vi "Monitor.vi"() -> ()   [LabVIEW 2015]
uses:
  Libraries/NI-DAQ/NI-DAQ digitizer parameters.ctl
  Libraries/File/Controls/File formats.ctl
panel:
  out "Shot data":string
  out "file path out":path
  out "Waveform Graph":waveform(dbl)[](graph)
  in  "Shots file":path=path "Y:/ShotHistory2016.txt"
  in  "Log file folder":path=path "C:/Data"
  out "Match out":errorcluster
  out "new path":path
  in  "Root Data Folder":path=path "C:/Data/idot"
  out "File count":i32
  out "New data file event":path
  out "Final error out":errorcluster
  out "Recorder Error Out":errorcluster
  in  "Parameters":T1={"physical channels"="Dev1/ai0:7", "input terminal configuration"=10106, "Range"=10.0, "Sample rate"=1000000.0, "samples per channel"=102400, "Trigger source"="/Dev1/PFI0", "pretrigger samples per channel"=1000, "task"="", "Sample mode"=10178, "Retriggerable"=FALSE, "File Path"=path "C:/Data/idot/test.tdms"} {"Sample mode" items=["Finite Samples"=10178, "Continuous Samples"=10123, "Hardware Timed Single Point"=12522]; "samples per channel" format="%d (0x%x)"; "Sample rate" format="%.2p"; "input terminal configuration" items=["default"=-1, "RSE"=10083, "NRSE"=10078, "Differential"=10106, "Pseudodifferential"=12529]}
  in  "Process Stop Button":bool
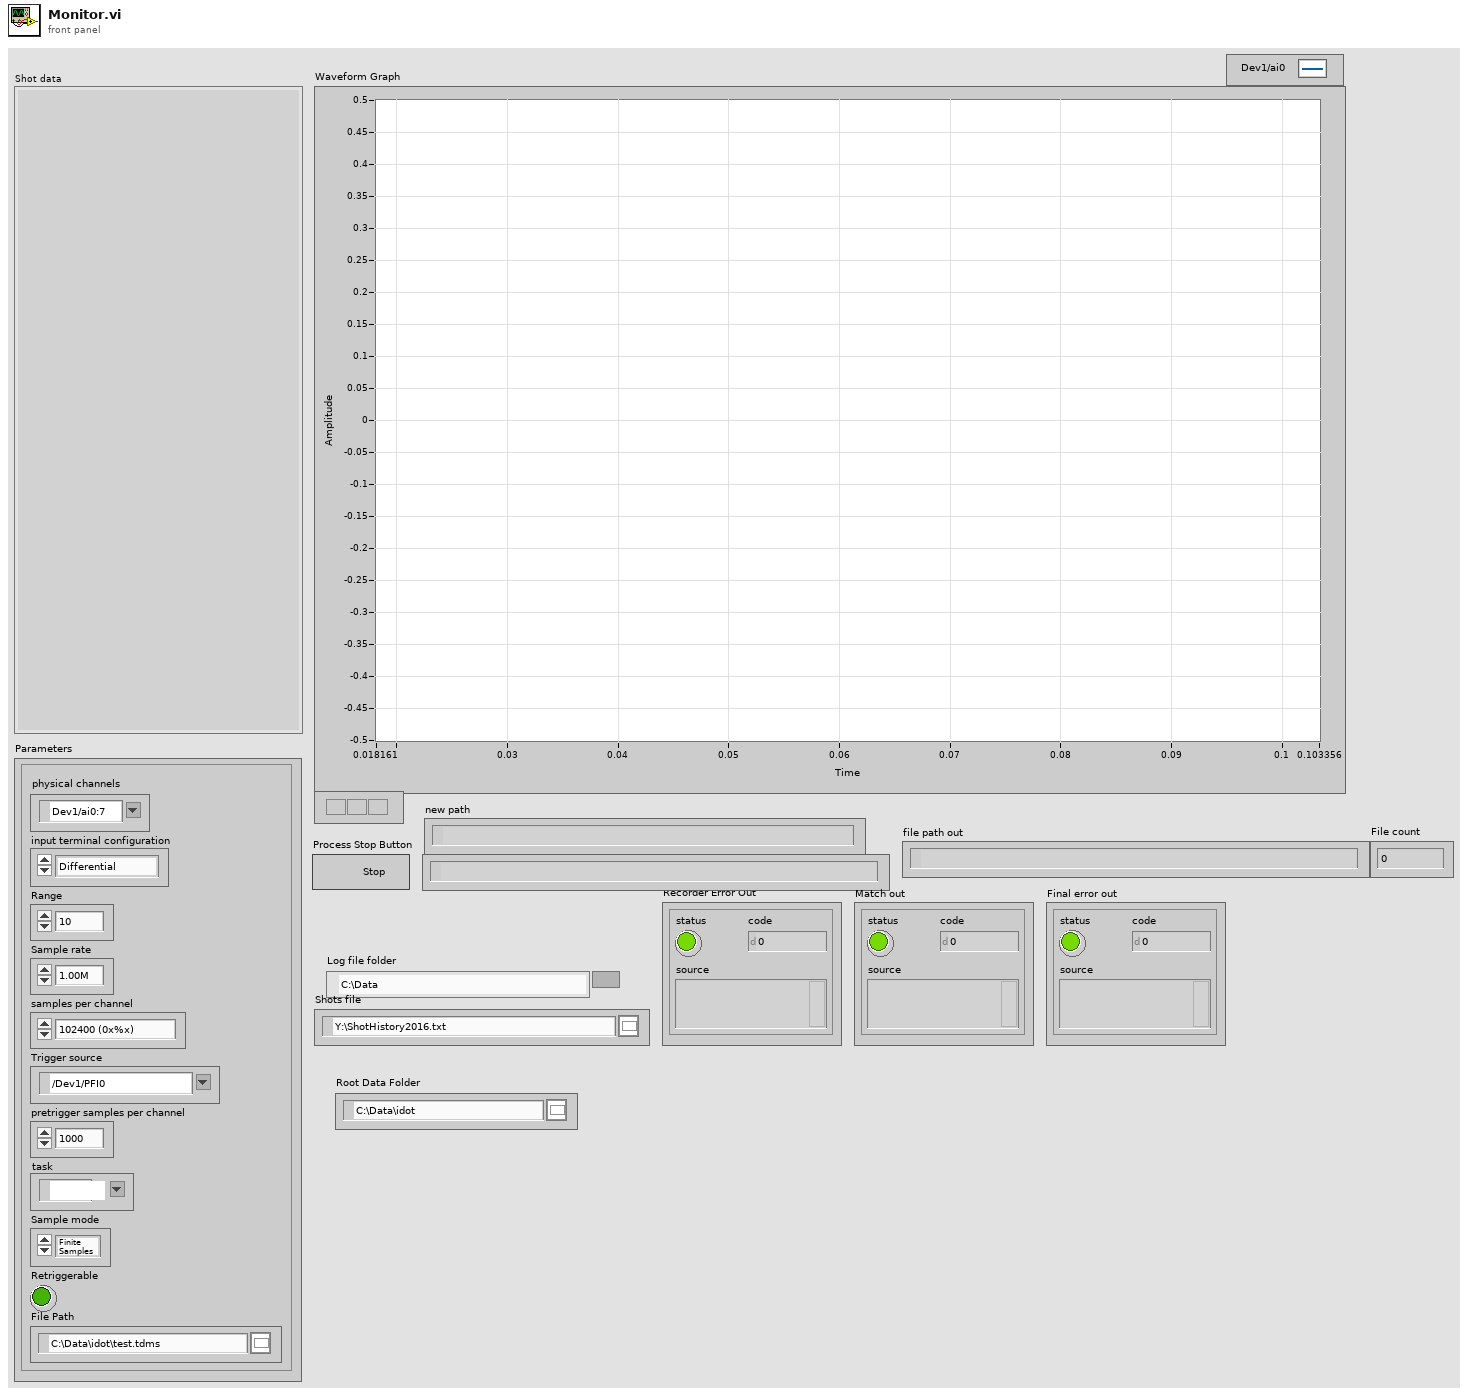
[diagram p1: front panel]
types:
  T1 = typedef "NI-DAQ digitizer parameters.ctl" = cluster{"physical channels":tag, "input terminal configuration":i32, "Range":dbl, "Sample rate":dbl, "samples per channel":i32, "Trigger source":tag, "pretrigger samples per channel":u32, "task":refnum<k21>, "Sample mode":i32, "Retriggerable":bool, "File Path":path}
  T2 = enum16{"open", "open or create", "create or replace", "create", "open (read-only)"}
  T3 = typedef "File formats.ctl" = enum16{"TDMS", "ASCII", "BINARY"}
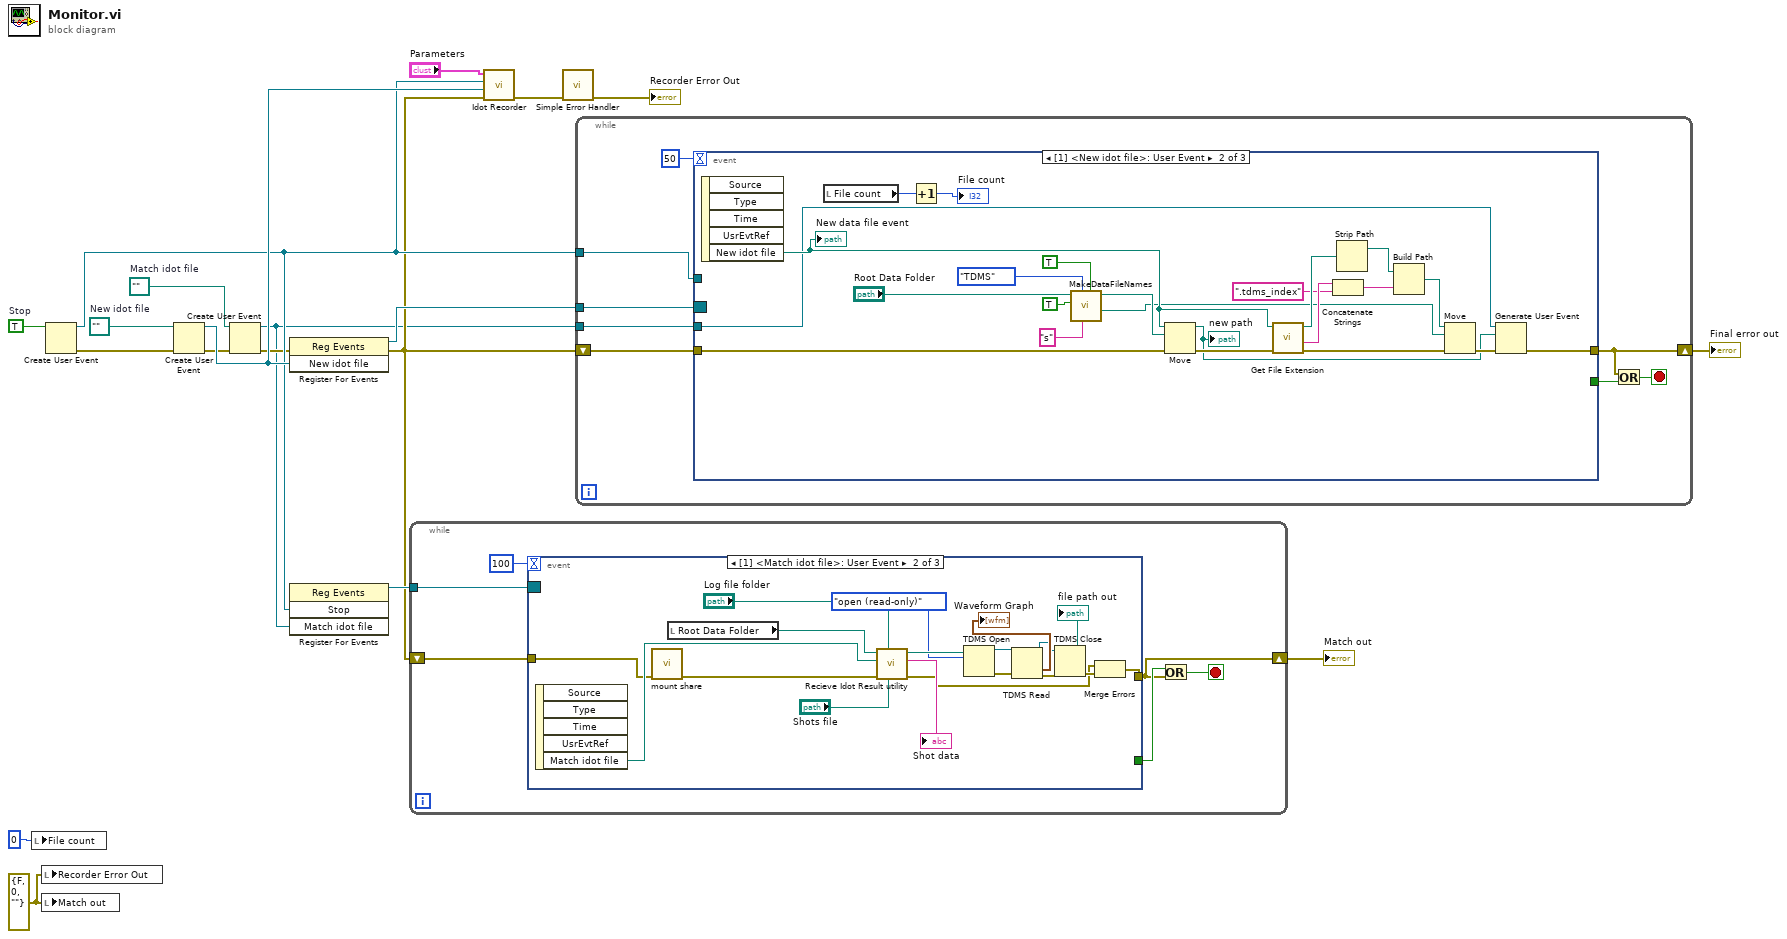
[diagram p0: block diagram]
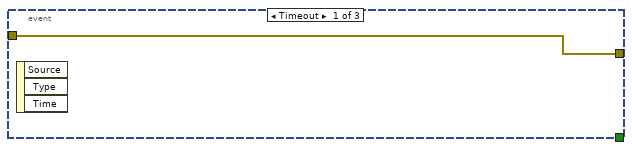
[diagram p2: hidden frame]
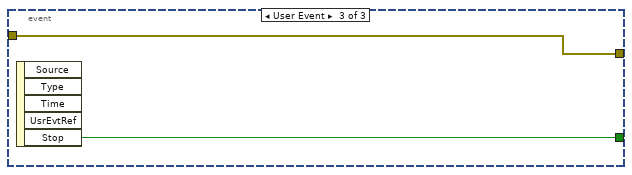
[diagram p3: hidden frame]
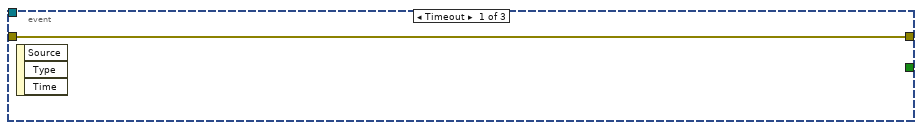
[diagram p4: hidden frame]
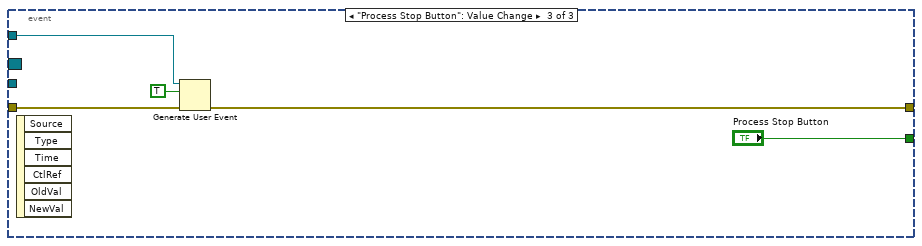
[diagram p5: hidden frame]
diagram:
  w6 = path ""  # Match idot file
  w2 = errorcluster {"status"=FALSE, "code"=0, "source"=""} ("Recorder Error Out")
  w18 = path ""  # New idot file
  w19 = TRUE  # Stop
  n1 = local write "File count"(0) -> ()
  n2 = local write "Recorder Error Out"(w2) -> ()
  n3 = local write "Match out"(w2) -> ()
  n4 = Create User Event(user event datatype=w19) -> (user event=w9:refnum<user-event>, error out=w16:errorcluster)  [unwired: 1 in]
  n5 = Create User Event(user event datatype=w18, error in=w16) -> (user event=w14:refnum<user-event>, error out=w8:errorcluster)
  n6 = Create User Event(user event datatype=w6, error in=w8) -> (user event=w1:refnum<user-event>, error out=w7:errorcluster)
  n7 = register-events(error in=w7, w14) -> (reference out=w13:refnum<event-registration>, error out=w4:errorcluster)  [unwired: 1 in]
  n8 = register-events(w9, w1) -> (reference out=w5:refnum<event-registration>)  [unwired: 2 in, 1 out]
  n9 = while {
    tunnel: w5 -> [w24]
    shift-right: [w20] -> w3
    shift-left: w4 -> [w22]
    stop <- w21 stop-if-true
    n10 = event shown="[1] <Match idot file>: User Event" {
      selector: w24 -> [_ _ _]
      dyn-events: _ -> [_ _ _]
      timeout: 100 -> [_ _ _]
      tunnel: [_ _ w46] -> w23
      tunnel: w22 -> [w26 w40 w45]
      tunnel: [w26 w28 w45] -> w20
      event Timeout {
        n11 = event-data() -> ()  [unwired: 1 in, 3 out]
      }
      event User Event {
        n12 = event-data() -> ("Match idot file"=w44:path)  [unwired: 1 in, 4 out]
        n13 = call "mount share.vi"("Error In"=w40) -> ("Error Out"=w39:errorcluster)  [unwired: 9 in, 1 out]
        n14 = local read "Root Data Folder"() -> (w43:path)
        n15 = call "Recieve Idot Result utility.vi"("Shots file"="Shots file", "Log file folder"="Log file folder", "error in (no error)"=w39, "file path"=w44, "Root Data Folder"=w43) -> ("error out"=w27:errorcluster, "Formated shot data"=→"Shot data":string, "File Path output"=w38:path)  [unwired: 4 in]
        n16 = TDMS Open(10:T2."open (read-only)" ("operation (0:open)"), 11:w38) -> (0:w35:errorcluster, 3:w36:refnum<k34>)  [unwired: 5 in]
        n17 = TDMS Read(0:w36, 11:w35) -> (4:w31:refnum<k34>, 10:→"Waveform Graph":waveform(dbl)[], 15:w33:errorcluster)  [unwired: 6 in, 3 out]
        n18 = TDMS Close(8:w33, 11:w31) -> (0:w32:errorcluster, 3:→"file path out":path)
        n19 = Merge Errors(w27, w32) -> (w28:errorcluster)
      }
      event User Event {
        n20 = event-data() -> ("Stop"=w46:bool)  [unwired: 1 in, 4 out]
      }
    }
    n21 = Or(x=w23, y=w20) -> (x .or. y?=w21:bool)
  }
  "Match out" <- w3
  n22 = call "Idot Recorder.vi"("Error In"=w4, "New idot file event"=w14, "Stop event"=w9, "Parameters"="Parameters") -> ("Error Out"=w15:errorcluster)  [unwired: 7 in]
  n23 = call <vilib>:"Simple Error Handler.vi"("error in (no error)"=w15) -> ("error out"=→"Recorder Error Out":errorcluster)  [unwired: 4 in, 4 out]
  n24 = while {
    tunnel: w13 -> [w53]
    shift-right: [w49] -> w12
    shift-left: w4 -> [w51]
    tunnel: w9 -> [w52]
    tunnel: w1 -> [w47]
    stop <- w50 stop-if-true
    n25 = event shown="[1] <New idot file>: User Event" {
      selector: w53 -> [_ _ _]
      dyn-events: _ -> [_ _ _]
      timeout: 50 -> [_ _ _]
      tunnel: [_ _ "Process Stop Button"] -> w54
      tunnel: w52 -> [_ _ w82]
      tunnel: w51 -> [w55 w70 w81]
      tunnel: [w55 w58 w80] -> w49
      tunnel: w47 -> [_ w57 _]
      event Timeout {
        n26 = event-data() -> ()  [unwired: 1 in, 3 out]
      }
      event User Event {
        n27 = event-data() -> ("New idot file"=w69:path)  [unwired: 1 in, 4 out]
        "New data file event" <- w69
        n28 = local read "File count"() -> (w77:i32)
        n29 = Increment(x=w77) -> (x+1=→"File count":i32)
        n30 = call "MakeDataFileNames.vi"("Include time"=TRUE, "File Prefix"="s", "File format"=File_formats."TDMS", "Generate Index"=TRUE, "Root Data Folder"="Root Data Folder") -> ("Index  File Path"=w60:path, "Data File  Path"=w71:path)  [unwired: 3 in, 2 out]
        n31 = Move(source path=w69, error in=w70, 10:w71) -> (error out=w63:errorcluster, 3:w56:path)  [unwired: 2 in, 1 out]
        "new path" <- w56
        n32 = call <vilib>:"Get File Extension.vi"("error in (no error)"=w63, "file"=w69) -> ("error out"=w62:errorcluster, "filename without extension"=w66:string, "dup file"=w68:path)  [unwired: 5 in, 2 out]
        n33 = Concatenate Strings(w66, ".tdms_index" ("string")) -> (w64:string)
        n34 = Strip Path(path=w68) -> (stripped path=w67:path)  [unwired: 1 out]
        n35 = Build Path(base path=w67, name or relative path=w64) -> (appended path=w61:path)
        n36 = Move(source path=w61, error in=w62, 10:w60) -> (error out=w59:errorcluster)  [unwired: 2 in, 2 out]
        n37 = Generate User Event(user event=w57, event data cluster=w56, error in=w59) -> (error out=w58:errorcluster)  [unwired: 1 in, 1 out]
      }
      event "Process Stop Button": Value Change {
        n38 = event-data() -> ()  [unwired: 1 in, 6 out]
        n39 = Generate User Event(user event=w82, event data cluster=TRUE ("event data"), error in=w81) -> (error out=w80:errorcluster)  [unwired: 1 in, 1 out]
      }
    }
    n40 = Or(x=w49, y=w54) -> (x .or. y?=w50:bool)
  }
  "Final error out" <- w12
